vi "ex3.vi"() -> ()   [LabVIEW 2018]
uses:
  <vilib>/Analysis/3filter.llb/Filter Passband Type.ctl
  <vilib>/Analysis/2dsp.llb/Real FFT.vi
  <vilib>/Analysis/3filter.llb/Butterworth Filter (DBL).vi
  <vilib>/measure/matone.llb/Extract Single Tone Information 1 Chan.vi
  <vilib>/Waveform/WDTOps.llb/WDT Append Waveforms DBL.vi
  <vilib>/Waveform/WDTOps.llb/WDT Waveform Duration DBL.vi
  <vilib>/Analysis/NI_AALPro.lvlib
  <vilib>/measure/NI_MAPro.lvlib
  <vilib>/Analysis/NI_AALBase.lvlib
panel:
  out "Waveform Graph 7":dbl[](graph)
  out "Waveform Graph 6":dbl[](graph)
  out "x-y":dbl
  out "Phase":dbl
  out "detected phase (deg)":dbl format="%.2p"
  out "Waveform Graph 5":dbl[](graph)
  out "arctan(x)":dbl
  out "Numeric 5":dbl format="%#_13g"
  out "Numeric 4":dbl format="%#_13g"
  out "Numeric 3":dbl format="%#_13g"
  out "x >= y? 3":bool
  out "x >= y? 2":bool
  out "x >= y?":bool
  out "duration":dbl format="%0.2f"
  out "size(s)":i32
  out "Numeric 2":dbl format="%#_13g"
  out "Numeric":dbl
  out "Array 4":dbl[](array[numeric])
  out "Array 3":dbl[](array[numeric])
  out "Array 2":dbl[](array[numeric])
  out "Array":dbl[](array[numeric])
  out "Waveform Graph 4":dynamicdata(graph)
  out "Waveform Graph 3":dynamicdata(graph)
  out "Waveform Graph 2":dynamicdata(graph)
  out "Waveform Graph":dynamicdata(graph)
  in  "stop (F)":bool
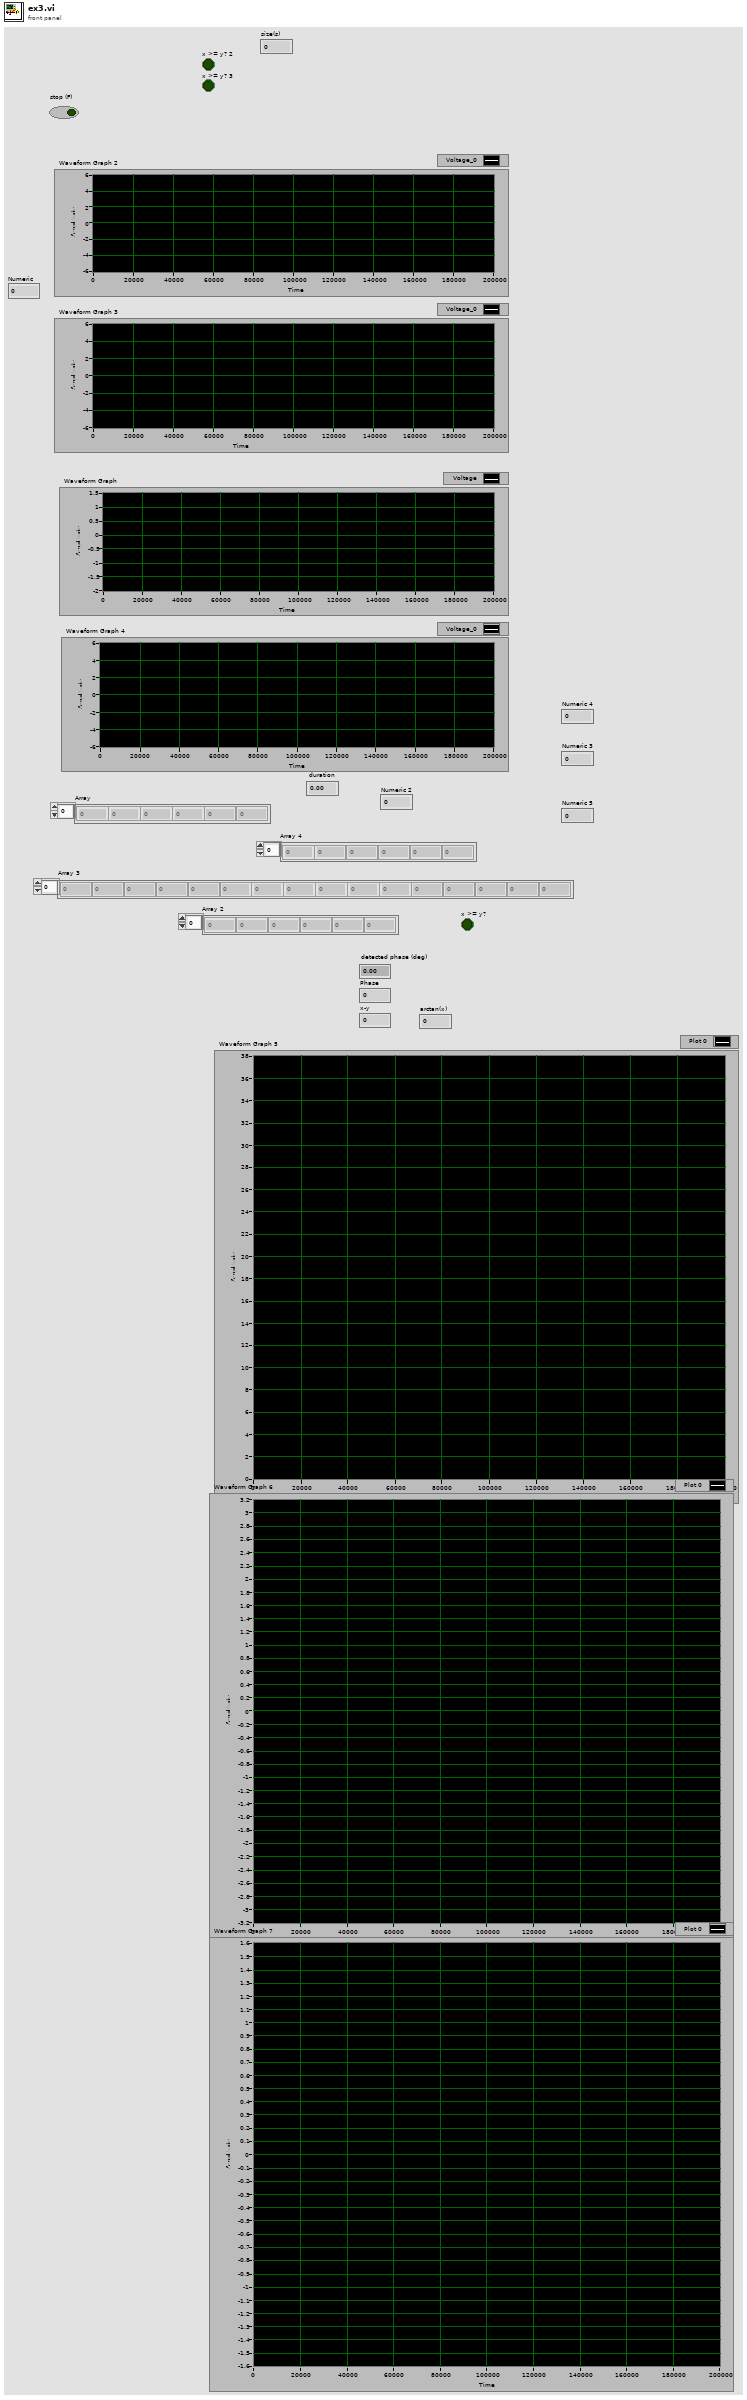
[diagram p1: front panel]
types:
  T1 = typedef "NI_AALBase.lvlib/Filter Passband Type.ctl" = enum32{"Lowpass", "Highpass", "Bandpass", "Bandstop"}
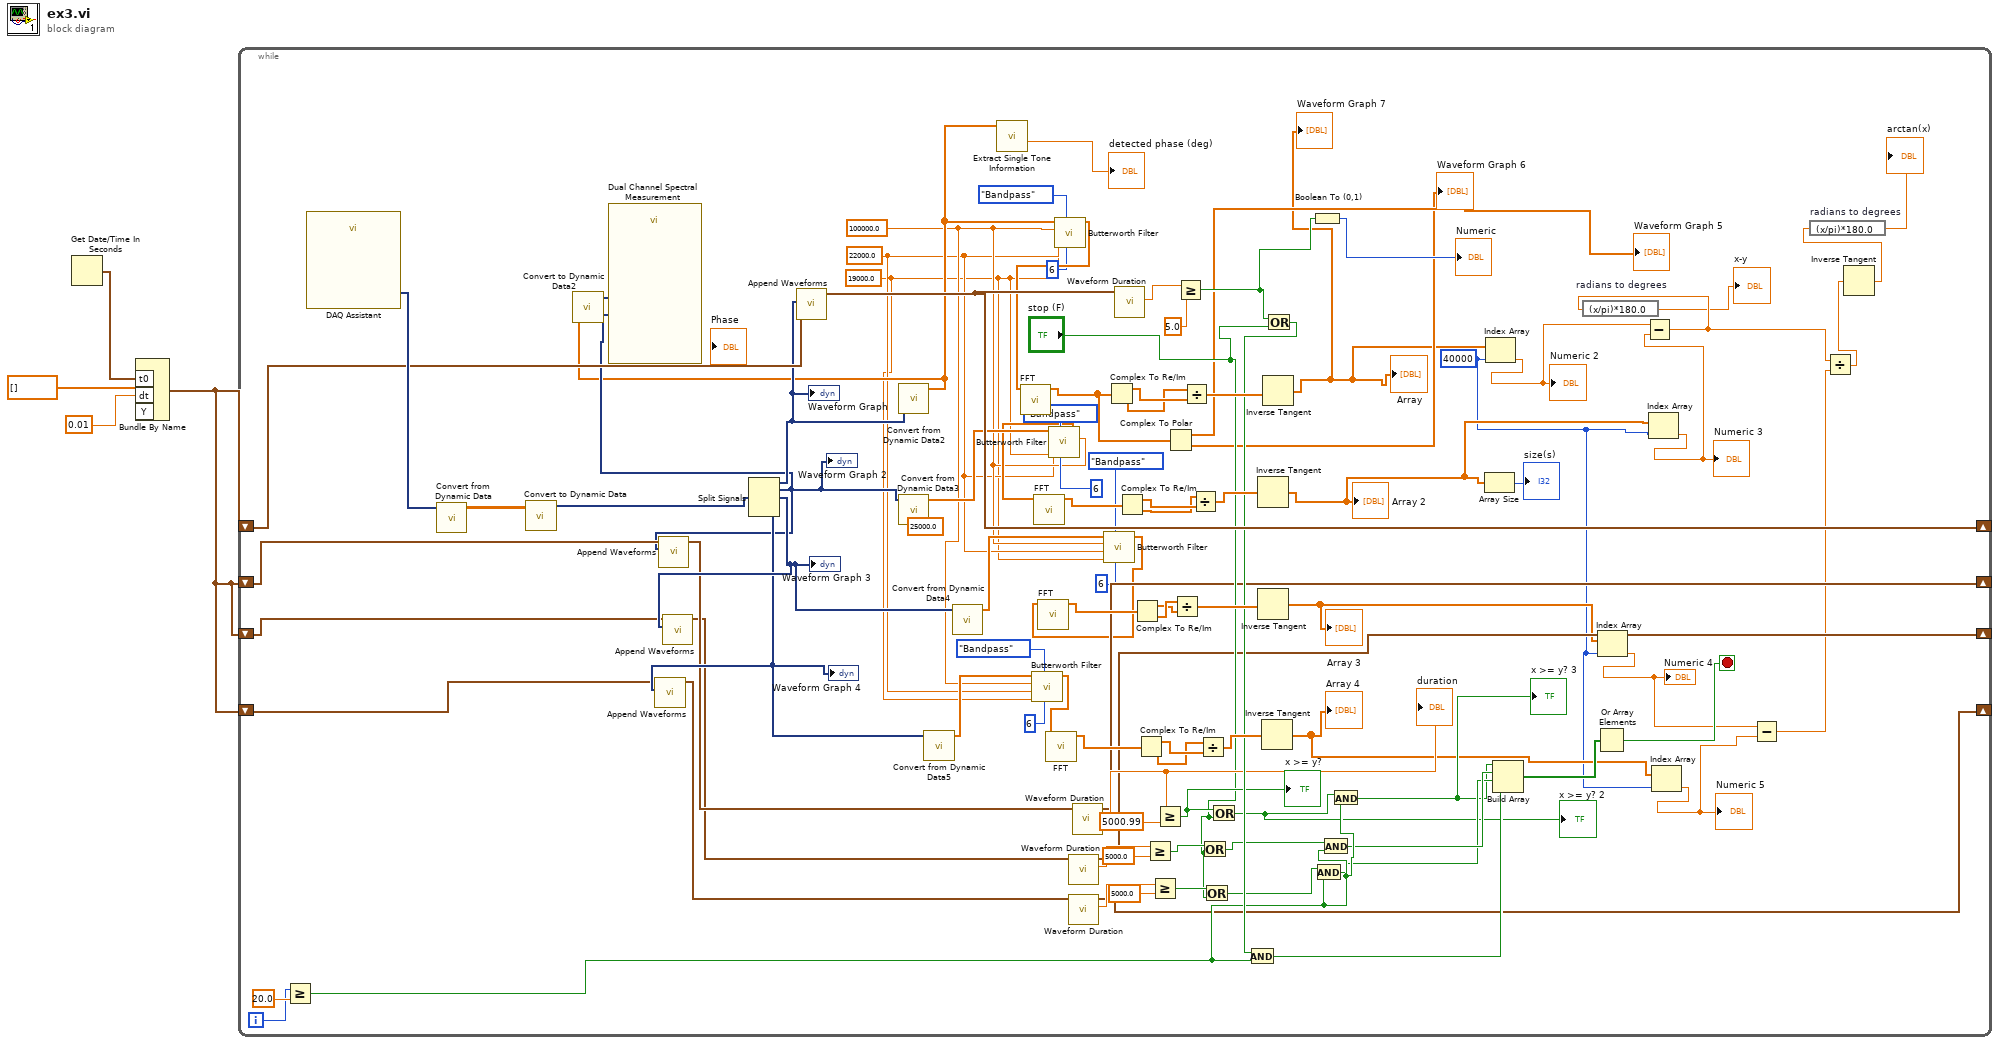
[diagram p0: block diagram]
diagram:
  n1 = Get Date/Time In Seconds() -> (seconds since 1Jan1904=w4:timestamp)
  n2 = Bundle By Name("t0"=w4, "dt"=0.01, "Y"=dbl[] []) -> (w1:waveform(dbl))  [unwired: 1 in]
  n3 = while {
    shift-right: [w89] -> _
    shift-left: w1 -> [w91]
    shift-right: [w58] -> _
    shift-left: w1 -> [w61]
    shift-right: [w57] -> _
    shift-left: w1 -> [w60]
    shift-right: [w56] -> _
    shift-left: w1 -> [w59]
    i -> [w87]
    stop <- w62 stop-if-true
    (unwired) 25000.0 ("low cutoff freq: fl")
    w8 = 19000.0 ("low cutoff freq: fl")
    w9 = 22000.0 ("high cutoff freq: fh")
    w10 = 100000.0 ("sampling freq: fs")
    w11 = 40000 ("index")
    n4 = Greater Or Equal?(x=w87, y=20.0) -> (x >= y?=w67:bool)
    n5 = call "DAQ Assistant"() -> ("data"=w97:dynamicdata)  [unwired: 16 in, 3 out]
    n6 = call "Convert from Dynamic Data"("Dynamic Data Type"=w97) -> ("Array"=w96:dbl[][])  [unwired: 3 in]
    n7 = call "Convert to Dynamic Data"("2D Array"=w96) -> ("Dynamic Data Type"=w90:dynamicdata)  [unwired: 3 in]
    n8 = Split Signals(w90) -> (w85:dynamicdata, w29:dynamicdata, w84:dynamicdata, w83:dynamicdata)  [unwired: 5 in, 1 out]
    "Waveform Graph" <- w85
    "Waveform Graph 2" <- w29
    "Waveform Graph 3" <- w84
    "Waveform Graph 4" <- w83
    n9 = call-poly <vilib>:"Append Waveforms.vi"("waveform B"=w83, "waveform A"=w59) -> ("waveform out"=w80:waveform(dbl))  [unwired: 8 in, 1 out]
    n10 = call-poly <vilib>:"Append Waveforms.vi"("waveform B"=w29, "waveform A"=w61) -> ("waveform out"=w82:waveform(dbl))  [unwired: 8 in, 1 out]
    n11 = call-poly <vilib>:"Append Waveforms.vi"("waveform B"=w84, "waveform A"=w60) -> ("waveform out"=w81:waveform(dbl))  [unwired: 8 in, 1 out]
    n12 = call-poly <vilib>:"Append Waveforms.vi"("waveform B"=w85, "waveform A"=w91) -> ("waveform out"=w89:waveform(dbl))  [unwired: 8 in, 1 out]
    n13 = call "Convert from Dynamic Data2"("Dynamic Data Type"=w85) -> ("Array"=w28:dbl[])  [unwired: 3 in]
    n14 = call "Convert to Dynamic Data2"("Array"=w28) -> ("Dynamic Data Type"=w32:dynamicdata)  [unwired: 3 in]
    n15 = call "Dual Channel Spectral Measurement"("Input Signal B"=w29, "Input Signal A"=w32) -> ()  [unwired: 7 in, 3 out]
    n16 = call "Convert from Dynamic Data3"("Dynamic Data Type"=w29) -> ("Array"=w13:dbl[])  [unwired: 3 in]
    n17 = call "Convert from Dynamic Data5"("Dynamic Data Type"=w83) -> ("Array"=w17:dbl[])  [unwired: 3 in]
    n18 = call "Convert from Dynamic Data4"("Dynamic Data Type"=w84) -> ("Array"=w15:dbl[])  [unwired: 3 in]
    n19 = call-poly <vilib>:"Extract Single Tone Information.vi"("time signal in"=w28) -> ("detected phase (deg)"=→"detected phase (deg)":dbl)  [unwired: 5 in, 5 out]
    n20 = call-poly <vilib>:"Butterworth Filter.vi"("order"=6, "filter type"=Filter_Passband_Type."Bandpass", "low cutoff freq: fl"=w8, "high cutoff freq: fh"=w9, "sampling freq: fs"=w10, "X"=w17) -> ("Filtered X"=w16:dbl[])  [unwired: 2 in, 1 out]
    n21 = call-poly <vilib>:"FFT.vi"("X"=w16) -> ("FFT {X}"=w102:cdb[])  [unwired: 9 in, 1 out]
    n22 = call-poly <vilib>:"Butterworth Filter.vi"("order"=6, "filter type"=Filter_Passband_Type."Bandpass", "low cutoff freq: fl"=w8, "high cutoff freq: fh"=w9, "sampling freq: fs"=w10, "X"=w13) -> ("Filtered X"=w12:dbl[])  [unwired: 2 in, 1 out]
    n23 = call-poly <vilib>:"FFT.vi"("X"=w12) -> ("FFT {X}"=w104:cdb[])  [unwired: 9 in, 1 out]
    n24 = call-poly <vilib>:"Butterworth Filter.vi"("order"=6, "filter type"=Filter_Passband_Type."Bandpass", "low cutoff freq: fl"=w8, "high cutoff freq: fh"=w9, "sampling freq: fs"=w10, "X"=w28) -> ("Filtered X"=w27:dbl[])  [unwired: 2 in, 1 out]
    n25 = call-poly <vilib>:"FFT.vi"("X"=w27) -> ("FFT {X}"=w34:cdb[])  [unwired: 9 in, 1 out]
    n26 = call-poly <vilib>:"Waveform Duration.vi"("waveform in"=w81) -> ("duration"=w77:dbl, "waveform out"=w57:waveform(dbl))  [unwired: 8 in, 1 out]
    n27 = call-poly <vilib>:"Waveform Duration.vi"("waveform in"=w80) -> ("duration"=w75:dbl, "waveform out"=w56:waveform(dbl))  [unwired: 8 in, 1 out]
    n28 = call-poly <vilib>:"Waveform Duration.vi"("waveform in"=w82) -> ("duration"=w79:dbl, "waveform out"=w58:waveform(dbl))  [unwired: 8 in, 1 out]
    "duration" <- w79
    n29 = call-poly <vilib>:"Butterworth Filter.vi"("order"=6, "filter type"=Filter_Passband_Type."Bandpass", "low cutoff freq: fl"=w8, "high cutoff freq: fh"=w9, "sampling freq: fs"=w10, "X"=w15) -> ("Filtered X"=w14:dbl[])  [unwired: 2 in, 1 out]
    n30 = call-poly <vilib>:"FFT.vi"("X"=w14) -> ("FFT {X}"=w103:cdb[])  [unwired: 9 in, 1 out]
    n31 = Complex To Re/Im(x + iy=w34) -> (x=w36:dbl[], y=w35:dbl[])
    n32 = call-poly <vilib>:"Waveform Duration.vi"("waveform in"=w89) -> ("duration"=w94:dbl)  [unwired: 8 in, 2 out]
    n33 = Complex To Re/Im(x + iy=w104) -> (x=w52:dbl[], y=w51:dbl[])
    n34 = Complex To Re/Im(x + iy=w103) -> (x=w49:dbl[], y=w50:dbl[])
    n35 = Complex To Re/Im(x + iy=w102) -> (x=w48:dbl[], y=w47:dbl[])
    n36 = Greater Or Equal?(x=w77, y=5000.0) -> (x >= y?=w72:bool)
    n37 = Greater Or Equal?(x=w75, y=5000.0) -> (x >= y?=w71:bool)
    n38 = Greater Or Equal?(x=w79, y=5000.99) -> (x >= y?=w73:bool)
    "x >= y?" <- w73
    n39 = Complex To Polar(r * e^(i*theta)=w34) -> (r=→"Waveform Graph 5":dbl[], theta=→"Waveform Graph 6":dbl[])
    n40 = Divide(x=w50, y=w49) -> (x/y=w100:dbl[])
    n41 = Greater Or Equal?(x=w94, y=5.0) -> (x >= y?=w93:bool)
    n42 = Divide(x=w35, y=w36) -> (x/y=w98:dbl[])
    n43 = Divide(x=w51, y=w52) -> (x/y=w99:dbl[])
    n44 = Divide(x=w47, y=w48) -> (x/y=w101:dbl[])
    n45 = Or(x=w72, y="stop (F)") -> (x .or. y?=w69:bool)
    n46 = Or(x=w71, y="stop (F)") -> (x .or. y?=w68:bool)
    n47 = Or(x=w73, y="stop (F)") -> (x .or. y?=w54:bool)
    "x >= y? 2" <- w54
    n48 = Inverse Tangent(1:w99) -> (0:w45:dbl[])
    "Array 2" <- w45
    n49 = Inverse Tangent(1:w100) -> (0:w46:dbl[])
    "Array 3" <- w46
    n50 = Inverse Tangent(1:w101) -> (0:w44:dbl[])
    "Array 4" <- w44
    n51 = Inverse Tangent(1:w98) -> (0:w5:dbl[])
    "Array" <- w5
    "Waveform Graph 7" <- w5
    n52 = Or(x=w93, y="stop (F)") -> (x .or. y?=w86:bool)
    n53 = And(x=w86, y=w67) -> (x .and. y?=w64:bool)
    n54 = Boolean To (0,1)(Boolean=w93) -> (0, 1=→"Numeric":i16)
    n55 = And(x=w68, y=w67) -> (x .and. y?=w65:bool)
    n56 = And(x=w69, y=w67) -> (x .and. y?=w66:bool)
    n57 = And(x=w54, y=w67) -> (x .and. y?=w53:bool)
    "x >= y? 3" <- w53
    n58 = Array Size(array=w45) -> (size(s)=→"size(s)":i32)
    n59 = Index Array(array=w5, index=w11) -> (element=w43:dbl)
    "Numeric 2" <- w43
    n60 = Build Array(w53, w66, w65, w64) -> (w63:bool[])
    n61 = Or Array Elements(Boolean array=w63) -> (logical OR=w62:bool)
    n62 = Index Array(array=w46, index=w11) -> (element=w40:dbl)
    "Numeric 4" <- w40
    n63 = Index Array(array=w45, index=w11) -> (element=w42:dbl)
    "Numeric 3" <- w42
    n64 = Subtract(x=w43, y=w42) -> (x-y=w31:dbl)
    n65 = expression code="(x/pi)*180.0" "radians to degrees"(w31) -> (→"x-y":dbl)
    n66 = Index Array(array=w44, index=w11) -> (element=w41:dbl)
    "Numeric 5" <- w41
    n67 = Subtract(x=w40, y=w41) -> (x-y=w39:dbl)
    n68 = Divide(x=w31, y=w39) -> (x/y=w38:dbl)
    n69 = Inverse Tangent(1:w38) -> (0:w37:dbl)
    n70 = expression code="(x/pi)*180.0" "radians to degrees"(w37) -> (→"arctan(x)":dbl)
  }
